vi "Get Position.vi"(8 "error in (no error)":errorcluster, 10 "Axis":i32=1, 11 "Abstract TranslationStage in":refnum<class "Abstract TranslationStage.lvclass">) -> (0 "error out":errorcluster, 1 "Position":dbl, 3 "Abstract TranslationStage out":refnum<class "Abstract TranslationStage.lvclass">)   [LabVIEW 2019, in "Abstract TranslationStage.lvclass"]
uses:
  Abstract TranslationStage.lvclass
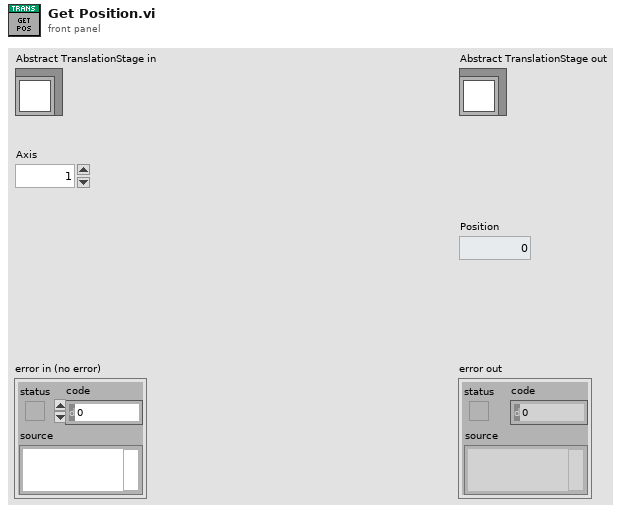
[diagram p1: front panel]
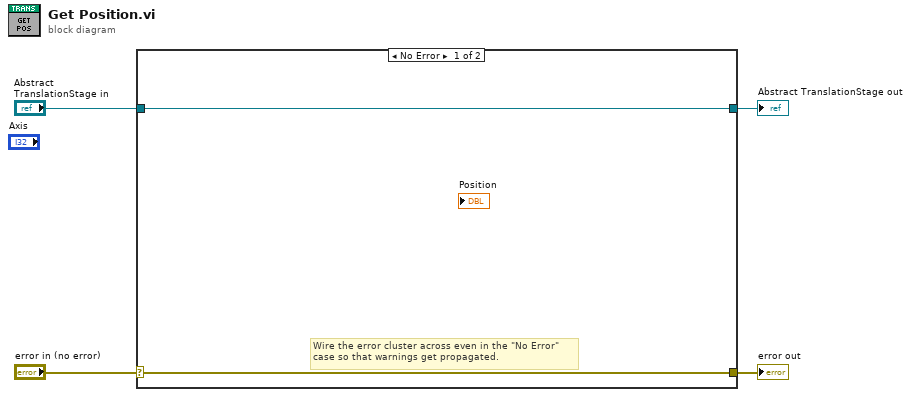
[diagram p0: block diagram]
diagram:
  n1 = case shown="No Error" "error in (no error)" {
    selector: "error in (no error)" -> [w5 w8]
    tunnel: [w5 w8] -> w3
    tunnel: [w6 w7] -> w1
    tunnel: "Abstract TranslationStage in" -> [w6 w7]
    frame No Error {
      # "Wire the error cluster across even in the \"No Error\"\ncase so that warnings get propagated."
    }
    frame Error {
    }
  }
  "error out" <- w3
  "Abstract TranslationStage out" <- w1
